vi "Data Logging.vi"   [LabVIEW 2016]
uses:
  Globale Variable/Globale Variable.vi
types:
  T1 = enum16{"open", "replace", "create", "open or create", "replace or create", "replace or create with confirmation"}
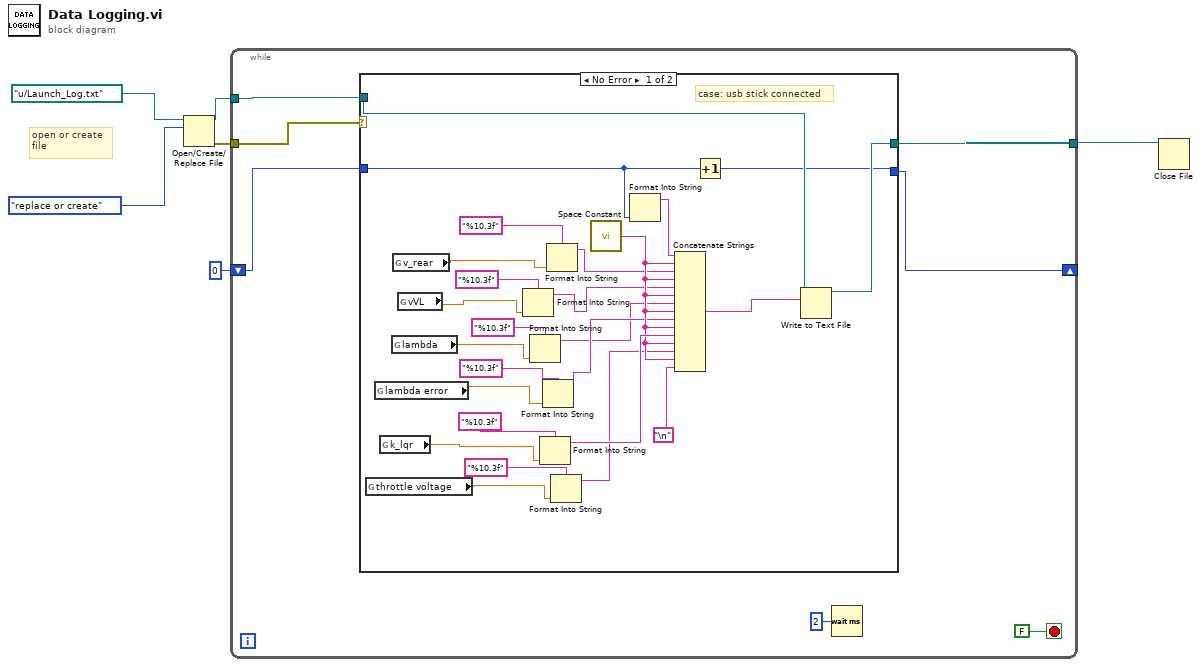
[diagram p0: block diagram]
diagram:
  # "open or create \nfile"
  n1 = Open/Create/Replace File(file path (use dialog)=path "u:/Launch_Log.txt", operation (0:open)=T1."replace or create") -> (refnum out=w4:refnum<file>, error out=w1:errorcluster)  [unwired: 4 in, 1 out]
  n2 = while {
    tunnel: w4 -> [w13]
    tunnel: [w12] -> w3
    shift-right: [w9] -> _
    shift-left: 0 -> [w10]
    tunnel: w1 -> [w8]
    stop <- FALSE stop-if-true
    n3 = case shown="No Error" w8 {
      tunnel: w13 -> [w37 w41]
      tunnel: [w39 w41] -> w12
      tunnel: w10 -> [w34 w40]
      tunnel: [w36 w40] -> w9
      frame No Error {
        # "case: usb stick connected"
        n4 = global read "Globale Variable.vi" "throttle voltage"() -> (w30:dbl)
        n5 = global read "Globale Variable.vi" "lambda error"() -> (w27:dbl)
        n6 = global read "Globale Variable.vi" "k_lqr"() -> (w32:dbl)
        n7 = global read "Globale Variable.vi" "lambda"() -> (w24:dbl)
        n8 = global read "Globale Variable.vi" "v_rear"() -> (w18:dbl)
        n9 = global read "Globale Variable.vi" "vVL"() -> (w21:dbl)
        n10 = Format Into String(format string="%10.3f", w21) -> (resulting string=w20:string)  [unwired: 2 in, 1 out]
        n11 = Format Into String(format string="%10.3f", w24) -> (resulting string=w23:string)  [unwired: 2 in, 1 out]
        n12 = Format Into String(format string="%10.3f", w32) -> (resulting string=w31:string)  [unwired: 2 in, 1 out]
        n13 = Format Into String(format string="%10.3f", w27) -> (resulting string=w26:string)  [unwired: 2 in, 1 out]
        n14 = Format Into String(format string="%10.3f", w18) -> (resulting string=w17:string)  [unwired: 2 in, 1 out]
        n15 = Format Into String(format string="%10.3f", w30) -> (resulting string=w15:string)  [unwired: 2 in, 1 out]
        n16 = call <vilib>:"Space Constant.vi"() -> ("String"=w28:string)
        n17 = Format Into String(w34) -> (resulting string=w35:string)  [unwired: 3 in, 1 out]
        n18 = Concatenate Strings(w35, w28, w17, w28, w20, w28, w23, w28, w26, w28, w31, w28, w15, w28, "\n") -> (w38:string)
        n19 = Increment(x=w34) -> (x+1=w36:i32)
        n20 = Write to Text File(file (use dialog)=w37, text=w38) -> (refnum out=w39:refnum<file>)  [unwired: 2 in, 2 out]
      }
      frame Error {
        # "case: no usb stick connected"
      }
    }
    n21 = Wait (ms)(milliseconds to wait=u32 2) -> ()  [unwired: 1 out]
  }
  n22 = Close File(refnum=w3) -> ()  [unwired: 1 in, 2 out]
